vi "Temperature Warnings.vi"(8 "Error In":errorcluster, 9 "Min Temperature":dbl, 10 "Max Temperature":dbl, 11 "Current Temperature":dbl) -> (0 "Error Out":errorcluster, 2 "Warning Text":string="No Warning", 3 "Warning?":bool)   [LabVIEW 2015]
doc: "This VI is used to determine the string to output to the weather station based on the current temperature and limit settings.\n\nInputs: Current Temperature (DBL), Minimum Temperature (DBL), and Maximum Temperature (DBL).\nOutputs: Warning Text (string) and Warning? (Boolean)."
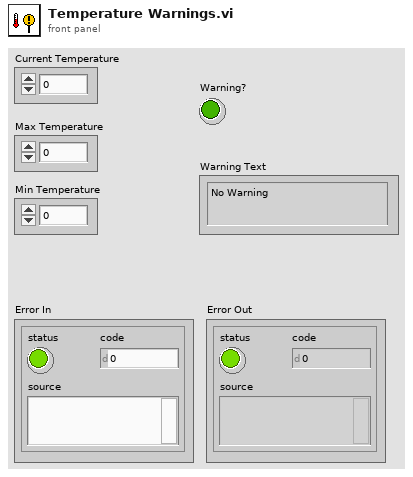
[diagram p1: front panel]
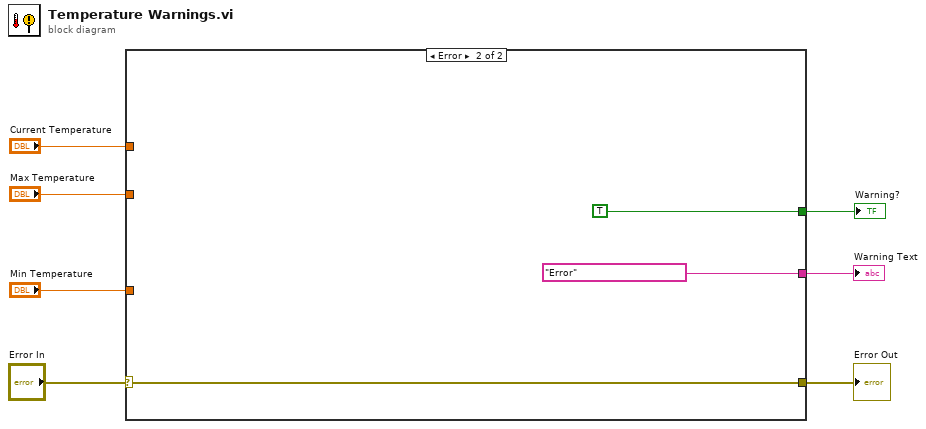
[diagram p0: block diagram]
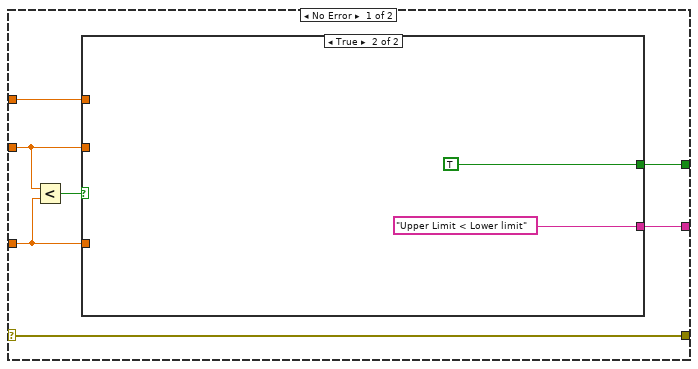
[diagram p2: hidden frame]
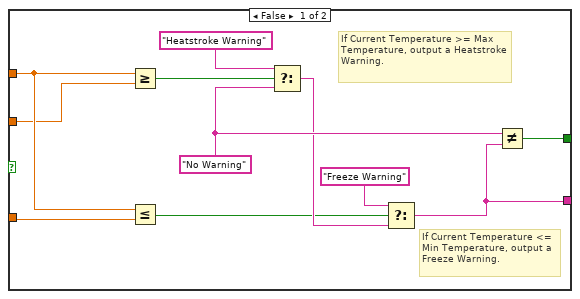
[diagram p3: hidden frame]
diagram:
  n1 = case shown="Error" "Error In" {
    selector: "Error In" -> [w14 w28]
    tunnel: [w14 w28] -> w6
    tunnel: [w13 TRUE] -> w5
    tunnel: [w12 "Error"] -> w4
    tunnel: "Current Temperature" -> [w11 _]
    tunnel: "Max Temperature" -> [w9 _]
    tunnel: "Min Temperature" -> [w8 _]
    frame No Error {
      n2 = Less?(x=w9, y=w8) -> (x < y?=w10:bool)
      n3 = case shown="True" w10 {
        tunnel: [w19 TRUE] -> w13
        tunnel: [w18 "Upper Limit < Lower limit"] -> w12
        tunnel: w11 -> [w17 _]
        tunnel: w9 -> [w16 _]
        tunnel: w8 -> [w15 _]
        frame False {
          w25 = "No Warning" ("f")
          # "If Current Temperature <= Min Temperature, output a Freeze Warning."
          # "If Current Temperature >= Max Temperature, output a Heatstroke Warning."
          n4 = Greater Or Equal?(x=w17, y=w16) -> (x >= y?=w20:bool)
          n5 = Less Or Equal?(x=w17, y=w15) -> (x <= y?=w23:bool)
          n6 = Select(t="Heatstroke Warning", s=w20, f=w25) -> (s? t:f=w24:string)
          n7 = Select(t="Freeze Warning", s=w23, f=w24) -> (s? t:f=w18:string)
          n8 = Not Equal?(x=w25, y=w18) -> (x != y?=w19:bool)
        }
        frame True {
        }
      }
    }
    frame Error {
    }
  }
  "Warning?" <- w5
  "Warning Text" <- w4
  "Error Out" <- w6
